vi "SE_HV200.destructor.vi"(0 "i ref in":refnum<vi>, 5 "error in(no error)":errorcluster) -> (19 "error out":errorcluster)   [LabVIEW 2014, in "SE_HV200.lvlib"]
doc: "This is the destructor of a class.\n\nLicense Agreement for this software:\n\nCopyright (C)\nGesellschaft für Schwerionenforschung, GSI\nPlanckstr. 1\n64291 Darmstadt\nGermany\n\nContact: D.Beck@gsi.de \n\nThis program is free software; you can redistribute it and/or modify it under the terms of the \nGNU General Public License as published by the Free Software Foundation; either version 2 of \nthe license, or (at your option) any later version.\n\nThis program is distributed in the hope that it will be useful, but WITHOUT ANY WARRANTY; \nwithout even the implied warranty of MERCHANTABILITY or FITNESS FOR A PARTICULAR PURPOSE. See the GNU General License for more details (http://www.gnu.org).\n\nGesellschaft für Schwerionenforschung, GSI\nPlanckstr. 1, 64291 Darmstadt, Germany\nFor all questions and ideas contact: M.Richter@gsi.de, H.Brand@gsi.de or D.Beck@gsi.de.\nLast update: 16-JUN-2004"
uses:
  SE_HV200.lvlib
  CSCore/BaseProcess/BaseProcess.lvlib
  CSlibraries-extern/DimLVEvent/LVDimInterface/LVDimInterface.lvlib
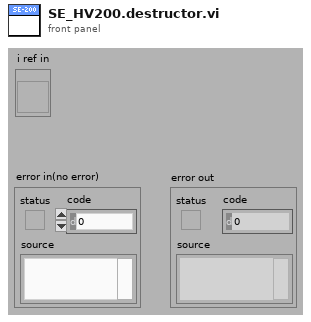
[diagram p1: front panel]
types:
  T1 = enum16{"SetAttribute", "GetAttribute", "CreateAttribute", "DestroyAttribute", "DestroyAllAtributes"}
  T2 = typedef "SE_HV200.lvlib/SE_HV200.i attribute.ctl" = cluster{"SetStatus":bool, "actVoltageID":i32, "VISA resource name in":refnum<visa-resource-name>, "Device name":string, "PSRange":i32, "nomVoltageID":i32, "actStatusID":i32, "NomVoltage":dbl[], "ActVoltage":dbl[], "DefaultChannel":i32}
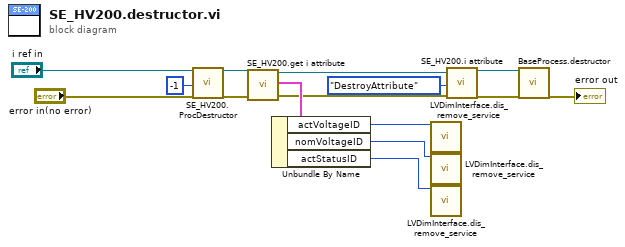
[diagram p0: block diagram]
diagram:
  n1 = call "SE_HV200.ProcDestructor.vi"("i ref in"="i ref in", "ms timeout (100)"=-1, "error in (no error)"="error in(no error)") -> ("i ref out"=w8:refnum<vi>, "error out"=w7:errorcluster)  [unwired: 14 in, 1 out]
  n2 = call "SE_HV200.get i attribute.vi"("i ref in"=w8, "error in (no error)"=w7) -> ("i ref out"=w5:refnum<vi>, "i attribute"=w6:T2, "error out"=w3:errorcluster)  [unwired: 15 in]
  n3 = Unbundle By Name(w6) -> ("actVoltageID"=w4:i32, "nomVoltageID"=w2:i32, "actStatusID"=w1:i32)
  n4 = call "LVDimInterface.dis_remove_service.vi"("my_serviceID"=w4) -> ()  [unwired: 18 in, 1 out]
  n5 = call "LVDimInterface.dis_remove_service.vi"("my_serviceID"=w2) -> ()  [unwired: 18 in, 1 out]
  n6 = call "LVDimInterface.dis_remove_service.vi"("my_serviceID"=w1) -> ()  [unwired: 18 in, 1 out]
  n7 = call "SE_HV200.i attribute.vi"("VI Refnum"=w5, "Action"=T1."DestroyAttribute", "error in (no error)"=w3) -> ("VI Refnum out"=w14:refnum<vi>, "error out"=w13:errorcluster)  [unwired: 14 in, 1 out]
  n8 = call "BaseProcess.destructor.vi"("i ref in"=w14, "error in (no error)"=w13) -> ("error out"=→"error out":errorcluster)  [unwired: 17 in]
